vi "Read File.vi"(10 "MXN":bool, 11 "Bakery Actor in":refnum<class "Bakery Actor.lvclass">) -> (2 "Array":string[][](array[string]), 3 "appended path":path)   [LabVIEW 2019, in "Bakery Actor.lvlib" / "Bakery Actor.lvclass"]
uses:
  Bakery Actor.lvclass
  <vilib>/Utility/config.llb/Read Key (Double).vi
  <vilib>/Utility/config.llb/Read Key (String).vi
  <vilib>/Utility/config.llb/NI_LVConfig.lvlib
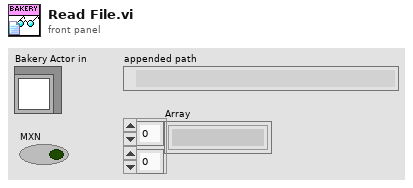
[diagram p1: front panel]
types:
  T1 = typedef "NI_LVConfig.lvlib/Config Data RefNum.ctl" = refnum<k1>
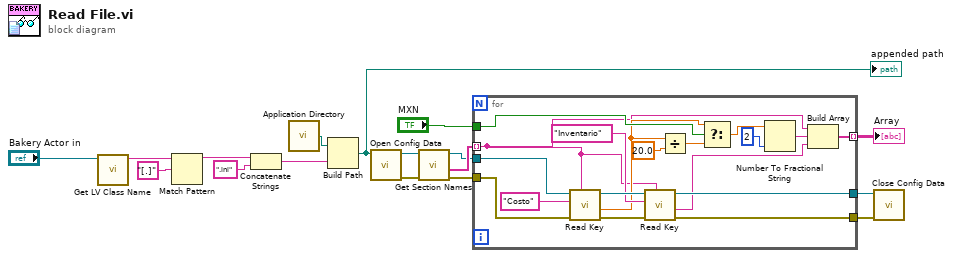
[diagram p0: block diagram]
diagram:
  n1 = call <vilib>:"Get LV Class Name.vi"("object"="Bakery Actor in") -> ("class name"=w7:string)  [unwired: 9 in, 1 out]
  n2 = Match Pattern(string=w7, regular expression="[.]") -> (before substring=w9:string)  [unwired: 1 in, 3 out]
  n3 = Concatenate Strings(w9, ".ini" ("string")) -> (w3:string)
  n4 = call <vilib>:"Application Directory.vi"() -> ("Application Directory"=w1:path)
  n5 = Build Path(base path=w1, name or relative path=w3) -> (appended path=w4:path)
  "appended path" <- w4
  n6 = call <vilib>:"Open Config Data.vi"("configuration file path"=w4) -> ("error out"=w12:errorcluster, "refnum"=w10:T1)  [unwired: 8 in, 1 out]
  n7 = call <vilib>:"Get Section Names.vi"("error in (no error)"=w12, "refnum"=w10) -> ("error out"=w13:errorcluster, "section names"=w14:string[], "refnum out"=w11:T1)  [unwired: 7 in]
  n8 = for {
    tunnel: w11 -> [w34]
    tunnel: w13 -> [w35]
    tunnel: [w31] -> w5
    tunnel: [w30] -> w6
    tunnel: w14 -> [w22] mode=indexing
    tunnel: "MXN" -> [w27]
    tunnel: [w19] -> w17 mode=indexing
    n9 = call-poly <vilib>:"Read Key.vi"("section"=w22, "error in (no error)"=w35, "key"="Costo" ("section"), "refnum"=w34) -> ("error out"=w33:errorcluster, "value"=w25:dbl, "refnum out"=w32:T1)  [unwired: 4 in, 1 out]
    n10 = call-poly <vilib>:"Read Key.vi"("section"=w22, "error in (no error)"=w33, "key"="Inventario" ("section"), "refnum"=w32) -> ("error out"=w31:errorcluster, "value"=w20:string, "refnum out"=w30:T1)  [unwired: 4 in, 1 out]
    n11 = Divide(x=w25, y=20.0) -> (x/y=w26:dbl)
    n12 = Select(t=w25, s=w27, f=w26) -> (s? t:f=w23:dbl)
    n13 = Number To Fractional String(number=w23, precision (6)=i16 2) -> (F-format string=w21:string)  [unwired: 2 in]
    n14 = Build Array(w22, w21, w20) -> (w19:string[])
  }
  "Array" <- w17
  n15 = call <vilib>:"Close Config Data.vi"("error in (no error)"=w5, "refnum"=w6) -> ()  [unwired: 8 in, 2 out]
